vi "Navigation_Main_r0.vi"() -> ()   [LabVIEW 2015]
uses:
  <vilib>/myRIO/Instrument Drivers/Onboard IO/PWM/typedefs/PWM Reference.ctl
  <vilib>/myRIO/Common/Instrument Driver Framework/Utilities/typedefs/myRIO Generic Hardware Reference.ctl
  <vilib>/myRIO/Common/Instrument Driver Framework/Utilities/typedefs/Hardware Version Enum.ctl
  <vilib>/myRIO/Common/Instrument Driver Framework/Utilities/typedefs/myRIO v1.0 Reference.ctl
  <vilib>/myRIO/Common/Instrument Driver Framework/Utilities/typedefs/Generic FPGA Reference.ctl
  <vilib>/myRIO/Common/Instrument Driver Framework/myRIO v1.0/PWM/typedefs/PWM Channels Enum.ctl
  <vilib>/myRIO/Instrument Drivers/Onboard IO/PWM/typedefs/PWM Configuration.ctl
  <vilib>/userdefined/High Color/nirio_resource_hc.ctl
  <vilib>/myRIO/Common/Instrument Driver Framework/myRIO v1.0/PWM/vis/myRIO v1.1 Open PWM.vi
  <vilib>/myRIO/Common/Instrument Driver Framework/Utilities/vis/Validate Channels.vi
  <vilib>/myRIO/Common/Instrument Driver Framework/myRIO v1.0/PWM/vis/myRIO v1.0 Reserve PWM.vi
  <vilib>/myRIO/Instrument Drivers/Onboard IO/PWM/vis/Set Duty Cycle and Frequency.vi
  <vilib>/myRIO/Common/Instrument Driver Framework/myRIO v1.0/PWM/vis/myRIO v1.0 Build MUX Configuration PWM.vi
  <vilib>/myRIO/Common/Instrument Driver Framework/myRIO v1.0/Resource Manager/vis/myRIO v1.0 Reserve Channel List.vi
  <vilib>/myRIO/Common/Instrument Driver Framework/myRIO v1.0/Resource Manager/vis/myRIO v1.0 Create Configuration List.vi
  <vilib>/myRIO/Common/Instrument Driver Framework/myRIO v1.0/Resource Manager/vis/myRIO v1.0 Reserve Channel.vi
  <vilib>/myRIO/Common/Instrument Driver Framework/myRIO v1.0/Resource Manager/vis/myRIO v1.0 Unreserve Channel.vi
  <vilib>/myRIO/Common/Instrument Driver Framework/myRIO v1.0/Resource Manager/vis/myRIO v1.0 Build Mutex Name.vi
  <vilib>/FPGAPlugInAG/myRIO-1900/niLvFpga_Open_myRIO-1900.vi
  <vilib>/rvi/interface/common/dynamic/niFpgaDynamicAddResources.vi
  <vilib>/myRIO/Common/Instrument Driver Framework/Utilities/vis/FPGA Ref Manager.vi
  <vilib>/Utility/error.llb/Error Cluster From Error Code.vi
  <vilib>/myRIO/Common/Instrument Driver Framework/Utilities/vis/Ref Counter.vi
  <vilib>/rvi/errors/niLvFpgaAdjustHostInterfaceError.vi
  <vilib>/Utility/VariantDataType/GetNumericInfo.vi
  <vilib>/myRIO/Common/Instrument Driver Framework/myRIO v1.0/myRIO v1.1 Open.vi
  <vilib>/myRIO/Common/Instrument Driver Framework/Utilities/vis/IO Manager.vi
  <vilib>/myRIO/Common/Instrument Driver Framework/Utilities/vis/Configuration Manager.vi
  <vilib>/myRIO/Common/Instrument Driver Framework/myRIO v1.0/Resource Manager/vis/myRIO v1.0 Configure IO.vi
  <vilib>/myRIO/Common/Instrument Driver Framework/myRIO v1.0/myRIO v1.0 Close.vi
  <vilib>/myRIO/Common/Instrument Driver Framework/myRIO v1.0/PWM/vis/myRIO v1.0 Write PWM.vi
  <vilib>/rvi/interface/nirviOpenFPGA/nirviOpenFPGA.xnode
  Navi/E/FPGA Bitfiles/NavigationProjec_FPGATarget2_FPGAMainNavigati_PWPHW8gwDxI.lvbitx
  <vilib>/rvi/interface/nirviReadWriteControl/nirviReadWriteControl.xnode
  <vilib>/myRIO/Instrument Drivers/Onboard IO/PWM/vis/myRIO PWM Open.xnode
  <vilib>/myRIO/Instrument Drivers/Onboard IO/PWM/PWM.lvlib
  <vilib>/myRIO/Instrument Drivers/Utilities/Utilities.lvlib
  NiFpgaLv.dll
  <vilib>/rvi/interface/Simulation/niFpgaSimulationCallBeginRW.vi
panel:
  out "left rear pwm":dbl
  out "left front pwm":dbl
  out "left mid pwm":dbl
  out "right rear pwm":dbl
  out "right mid pwm":dbl
  out "right front pwm":dbl
  in  "Full Ahead Captain":bool
  out "LF Rot Velocity (rot/s)":dbl
  out "LM Rot Velocity (rot/s)":dbl
  out "LR Rot Velocity (rot/s)":dbl
  in  "All Left Enable":bool
  in  "All Right Enable":bool
  out "RR Rot Velocity (rot/s)":dbl
  out "RM Linear Velocity (rot/s)":dbl
  out "RF Linear Velocity (rot/s)":dbl
  in  "Auto?":bool
  in  "Encoder Reset":bool
  out "L Min Linear Velocity (ft/s) 2":dbl
  out "R Min Linear Velocity (ft/s)  2":dbl
  in  "Goal Y":dbl=3.0 format="%#_13g"
  in  "Goal X":dbl=20.0 format="%#_13g"
  out "x+y":dbl
  in  "Current Y Pos":dbl=5.0 format="%#_13g"
  in  "Current X Pos":dbl=20.0 format="%#_13g"
  out "SYS.SELECTA":u8 format="%08b"
  out "ENC.B_c.CNTR":i32
  out "ENC.B_b.CNTR":i32
  out "ENC.B_a.CNTR":i32
  out "ENC.A_c.CNTR":i32
  out "ENC.A_b.CNTR":i32
  out "ENC.A_a.CNTR":i32
  out "Toggle \nIndicator":bool
  in  "R Desired Input Velocity (ft/s) 2":dbl(knob) scale=-4.0..4.0
  in  "Right Front Enable":bool
  in  "Right Mid Enable":bool
  in  "Right Rear Enable":bool
  in  "Left front enable":bool
  in  "Left mid enable":bool
  in  "Left rear enable":bool
  in  "Sync L -> R":bool
  in  "R Min Linear Velocity (ft/s)":dbl=-2.0 format="%#_13g"
  in  "R Max Linear Velocity (ft/s)":dbl=2.0 format="%#_13g"
  in  "L Min Linear Velocity (ft/s)":dbl=-2.0 format="%#_13g"
  in  "L Max Linear Velocity (ft/s)":dbl=2.0 format="%#_13g"
  out "Current Rot Velocity (rot/s)":T1(graph)
  in  "L Desired Input Velocity (ft/s)":dbl(knob) scale=-4.0..4.0
  # "Motor Control Parameters"
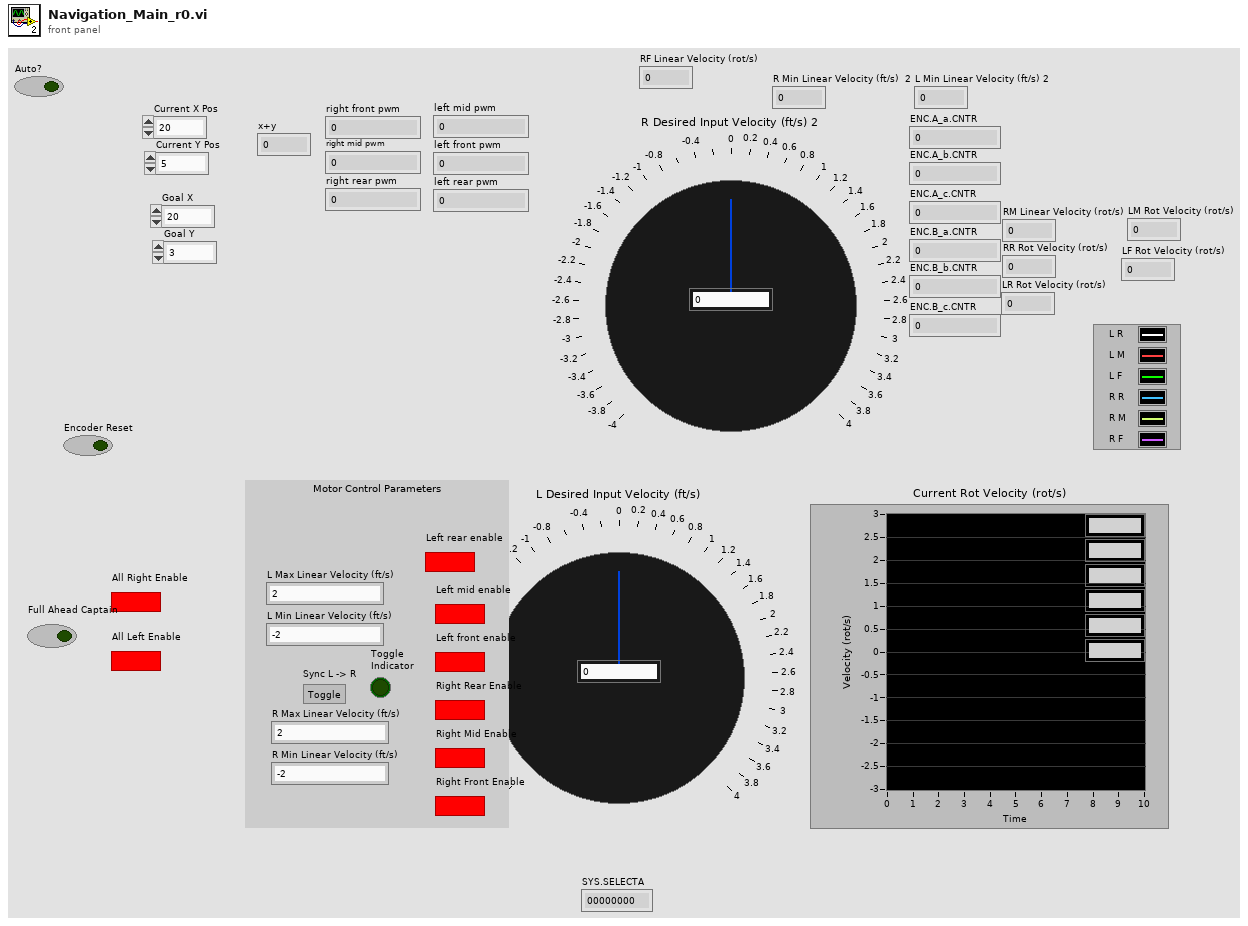
[diagram p1: front panel]
types:
  T1 = cluster{"Rotational Velocity (RPS)":dbl, "Rotational Velocity (RPS)":dbl, "Rotational Velocity (RPS)":dbl, "Rotational Velocity (RPS)":dbl, "Rotational Velocity (RPS)":dbl, "Rotational Velocity (RPS)":dbl}
  T2 = typedef "nirio_resource_hc.ctl" = tag
  T3 = typedef "Hardware Version Enum.ctl" = enum16{"Unknown", "myRIO-1900", "myRIO-1950", "roboRIO"}
  T4 = typedef "PWM.lvlib/PWM Reference.ctl" = cluster{"myRIO Reference":T5, "PWM Channels Enum":T8, "PWM Configuration":T9}
  T5 = typedef "myRIO Generic Hardware Reference.ctl" = cluster{"myRIO Model":T3, "myRIO Hardware Reference":T6}
  T6 = typedef "myRIO v1.0 Reference.ctl" = cluster{"Generic FPGA Reference":T7, "Allow multiple opens":bool}
  T7 = typedef "Generic FPGA Reference.ctl" = refnum<k20>
  T8 = typedef "PWM Channels Enum.ctl" = enum16{"Not Connected", "C/PWM0", "C/PWM1", "A/PWM0", "A/PWM1", "A/PWM2", "B/PWM0", "B/PWM1", "B/PWM2", "PWM/PWM0", "PWM/PWM1", "PWM/PWM2", "PWM/PWM3", "PWM/PWM4", "PWM/PWM5", "PWM/PWM6", "PWM/PWM7", "PWM/PWM8", "PWM/PWM9"}
  T9 = typedef "PWM.lvlib/PWM Configuration.ctl" = cluster{"Frequency":dbl, "Duty Cycle":dbl}
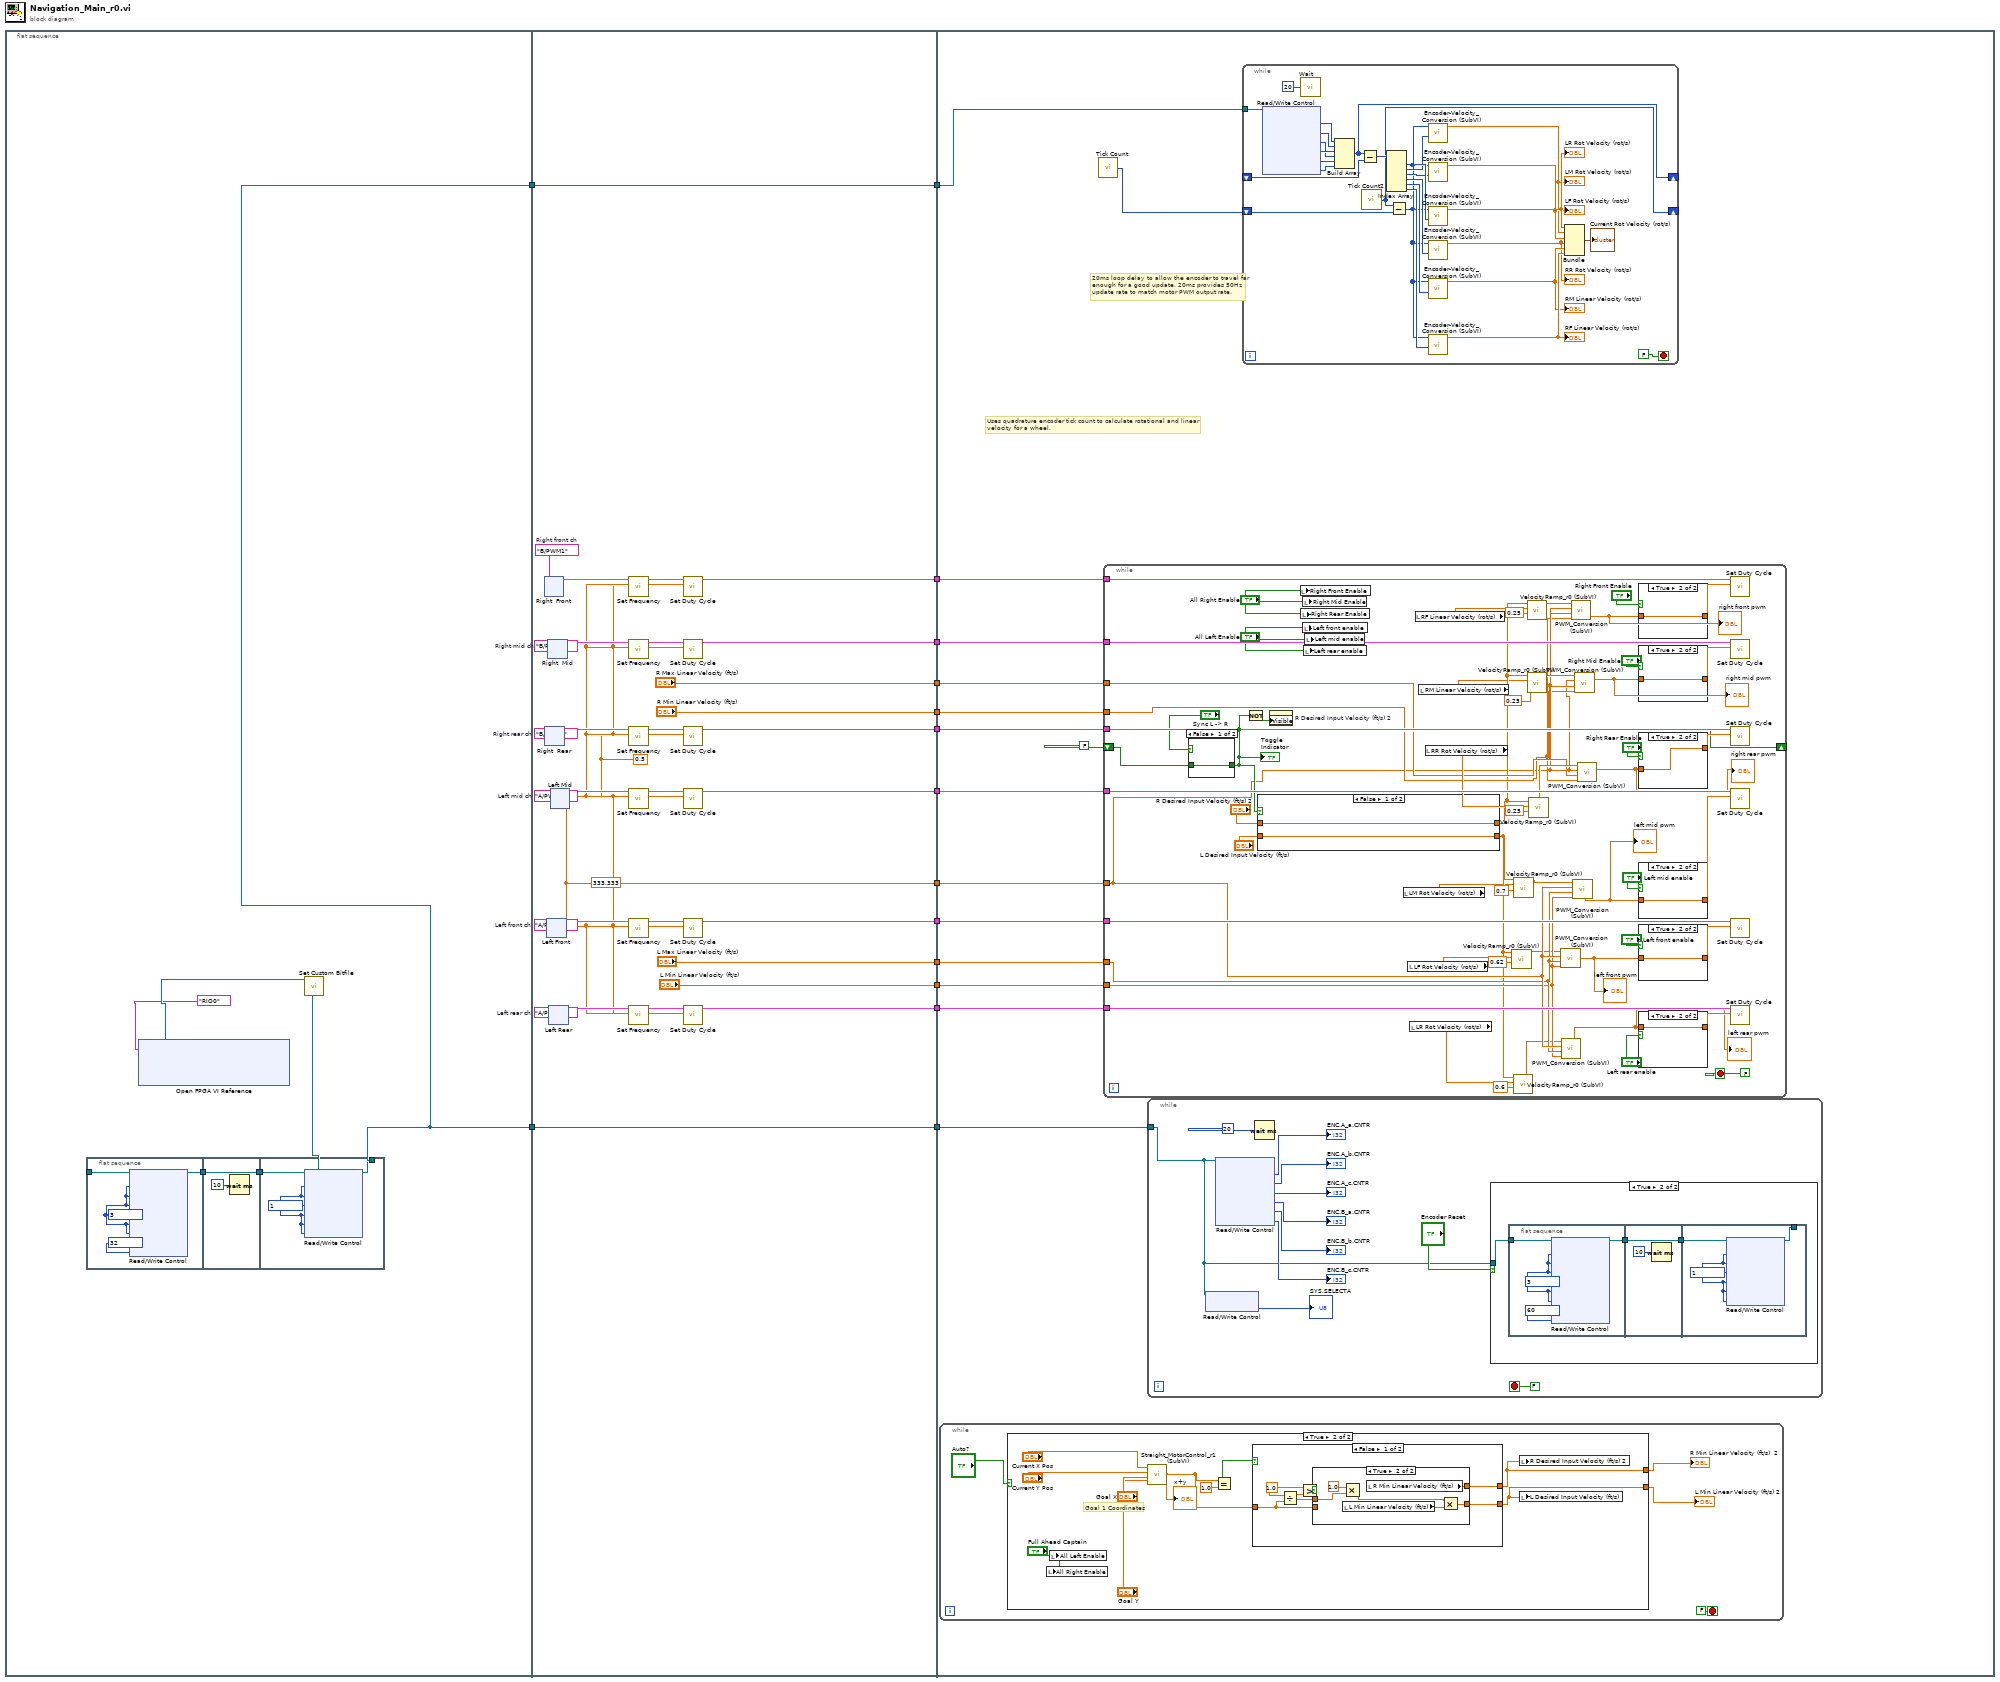
[diagram p0: block diagram]
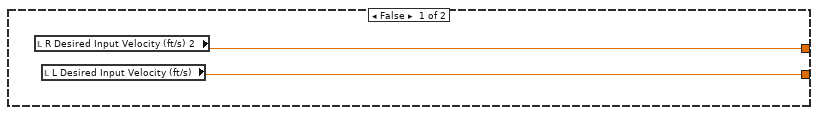
[diagram p2: hidden frame]
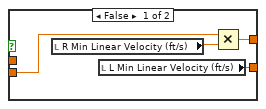
[diagram p3: hidden frame]
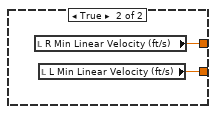
[diagram p4: hidden frame]
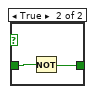
[diagram p6: hidden frame]
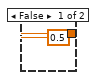
[diagram p7: hidden frame]
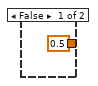
[diagram p8: hidden frame]
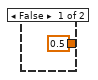
[diagram p9: hidden frame]
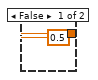
[diagram p10: hidden frame]
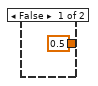
[diagram p11: hidden frame]
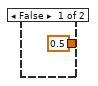
[diagram p12: hidden frame]
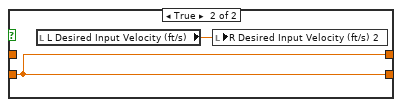
[diagram p13: hidden frame]
diagram:
  n1 = flat-sequence {
    tunnel: [w18] -> w3
    tunnel: [w18] -> w1
    tunnel: [w50] -> w15
    tunnel: [w45] -> w14
    tunnel: [w41] -> w13
    tunnel: [w40] -> w12
    tunnel: [w39] -> w11
    tunnel: [w38] -> w10
    tunnel: [w37] -> w9
    tunnel: ["L Max Linear Velocity (ft/s)"] -> w8
    tunnel: ["L Min Linear Velocity (ft/s)"] -> w7
    tunnel: ["R Max Linear Velocity (ft/s)"] -> w6
    tunnel: ["R Min Linear Velocity (ft/s)"] -> w5
    tunnel: [w32] -> w4
    tunnel: w3 -> [w31]
    tunnel: [w31] -> w2
    tunnel: w1 -> [w32]
    tunnel: w15 -> [w172]
    tunnel: w14 -> [w171]
    tunnel: w13 -> [w170]
    tunnel: w12 -> [w169]
    tunnel: w11 -> [w168]
    tunnel: w10 -> [w167]
    tunnel: w9 -> [w166]
    tunnel: w8 -> [w165]
    tunnel: w7 -> [w164]
    tunnel: w6 -> [w163]
    tunnel: w5 -> [w162]
    tunnel: w4 -> [w160]
    tunnel: w2 -> [w159]
    frame #0 {
      n2 = flat-sequence {
        tunnel: w19 -> [w24]
        tunnel: [w22] -> w21
        tunnel: w21 -> [w26]
        tunnel: [w26] -> w20
        tunnel: w20 -> [w29]
        tunnel: [w28] -> w18
        frame #0 {
          w23 = u8 32 ("SYS.SELECTA")
          w25 = u8 3 ("ENC.B_c.CNFG")
          n3 = xnode "Read/Write Control"("FPGA VI Reference In"=w24, "ENC.A_a.CNFG"=w25, "ENC.A_b.CNFG"=w25, "ENC.A_c.CNFG"=w25, "ENC.B_a.CNFG"=w25, "ENC.B_b.CNFG"=w25, "ENC.B_c.CNFG"=w25, "SYS.SELECTA"=w23, "SYS.SELECTB"=w23) -> ("FPGA VI Reference Out"=w22:refnum<k20>)  [unwired: 1 in, 1 out]
        }
        frame #1 {
          n4 = Wait (ms)(milliseconds to wait=u32 10) -> ()  [unwired: 1 out]
        }
        frame #2 {
          w30 = u8 1 ("ENC.B_c.CNFG")
          n5 = xnode "Read/Write Control"("FPGA VI Reference In"=w29, "ENC.A_a.CNFG"=w30, "ENC.A_b.CNFG"=w30, "ENC.A_c.CNFG"=w30, "ENC.B_a.CNFG"=w30, "ENC.B_b.CNFG"=w30, "ENC.B_c.CNFG"=w30) -> ("FPGA VI Reference Out"=w28:refnum<k20>)  [unwired: 1 in, 1 out]
        }
      }
      n6 = xnode "Open FPGA VI Reference"("resource name"=tag "RIO0") -> ("FPGA VI Reference Out"=w17:refnum<k20>)  [unwired: 1 in, 1 out]
      n7 = call <vilib>:"Set Custom Bitfile.vi"("Custom FPGA Reference In"=w17) -> ("Custom FPGA Reference Out"=w19:refnum<k20>)  [unwired: 9 in, 1 out]
    }
    frame #1 {
      w42 = 0.5 ("Duty Cycle")
      w50 = 333.333 ("Frequency [Hz]")
      w57 = tag "B/PWM2"  # Right rear ch
      w58 = tag "B/PWM0"  # Right mid ch
      w59 = tag "B/PWM1"  # Right front ch
      w60 = tag "A/PWM2"  # Left rear ch
      w61 = tag "A/PWM1"  # Left mid ch
      w62 = tag "A/PWM0"  # Left front ch
      n8 = xnode "Right  Front"("Channel Name"=w59) -> ("PWM Ref Out"=w53:T4)  [unwired: 2 in, 1 out]
      n9 = xnode "Right  Rear"("Channel Name"=w57) -> ("PWM Ref Out"=w51:T4)  [unwired: 2 in, 1 out]
      n10 = xnode "Left Front"("Channel Name"=w62) -> ("PWM Ref Out"=w56:T4)  [unwired: 2 in, 1 out]
      n11 = xnode "Right  Mid"("Channel Name"=w58) -> ("PWM Ref Out"=w52:T4)  [unwired: 2 in, 1 out]
      n12 = xnode "Left Rear"("Channel Name"=w60) -> ("PWM Ref Out"=w54:T4)  [unwired: 2 in, 1 out]
      n13 = xnode "Left Mid"("Channel Name"=w61) -> ("PWM Ref Out"=w55:T4)  [unwired: 2 in, 1 out]
      n14 = call <vilib>:"Set Frequency.vi"("Frequency [Hz]"=w50, "PWM Ref In"=w53) -> ("PWM Ref Out"=w46:T4)  [unwired: 7 in, 1 out]
      n15 = call <vilib>:"Set Frequency.vi"("Frequency [Hz]"=w50, "PWM Ref In"=w52) -> ("PWM Ref Out"=w47:T4)  [unwired: 7 in, 1 out]
      n16 = call <vilib>:"Set Frequency.vi"("Frequency [Hz]"=w50, "PWM Ref In"=w51) -> ("PWM Ref Out"=w48:T4)  [unwired: 7 in, 1 out]
      n17 = call <vilib>:"Set Frequency.vi"("Frequency [Hz]"=w50, "PWM Ref In"=w55) -> ("PWM Ref Out"=w43:T4)  [unwired: 7 in, 1 out]
      n18 = call <vilib>:"Set Frequency.vi"("Frequency [Hz]"=w50, "PWM Ref In"=w56) -> ("PWM Ref Out"=w49:T4)  [unwired: 7 in, 1 out]
      n19 = call <vilib>:"Set Frequency.vi"("Frequency [Hz]"=w50, "PWM Ref In"=w54) -> ("PWM Ref Out"=w44:T4)  [unwired: 7 in, 1 out]
      n20 = call <vilib>:"Set Duty Cycle.vi"("Duty Cycle"=w42, "PWM Ref In"=w46) -> ("PWM Ref Out"=w41:T4)  [unwired: 7 in, 1 out]
      n21 = call <vilib>:"Set Duty Cycle.vi"("Duty Cycle"=w42, "PWM Ref In"=w47) -> ("PWM Ref Out"=w40:T4)  [unwired: 7 in, 1 out]
      n22 = call <vilib>:"Set Duty Cycle.vi"("Duty Cycle"=w42, "PWM Ref In"=w48) -> ("PWM Ref Out"=w39:T4)  [unwired: 7 in, 1 out]
      n23 = call <vilib>:"Set Duty Cycle.vi"("Duty Cycle"=w42, "PWM Ref In"=w43) -> ("PWM Ref Out"=w38:T4)  [unwired: 7 in, 1 out]
      n24 = call <vilib>:"Set Duty Cycle.vi"("Duty Cycle"=w42, "PWM Ref In"=w49) -> ("PWM Ref Out"=w37:T4)  [unwired: 7 in, 1 out]
      n25 = call <vilib>:"Set Duty Cycle.vi"("Duty Cycle"=w42, "PWM Ref In"=w44) -> ("PWM Ref Out"=w45:T4)  [unwired: 7 in, 1 out]
    }
    frame #2 {
      # "Uses quadrature encoder tick count to calculate rotational and linear velocity for a wheel."
      # "20ms loop delay to allow the encoder to travel far enough for a good update. 20ms provides 50Hz update rate to match motor PWM output rate."
      n26 = while {
        stop <- FALSE stop-if-true
        n27 = case shown="True" "Auto?" {
          tunnel: [w178 w181] -> w176
          tunnel: [w179 w182] -> w175
          frame False {
            n28 = local read "R Desired Input Velocity (ft/s) 2"() -> (w178:dbl)
            n29 = local read "L Desired Input Velocity (ft/s)"() -> (w179:dbl)
          }
          frame True {
            # "Goal 1 Coordinates"
            n30 = local write "All Right Enable"("Full Ahead Captain") -> ()
            n31 = local write "All Left Enable"("Full Ahead Captain") -> ()
            n32 = call "Straight_MotorControl_r1 (SubVI).vi"("Goal Y Coord"="Goal Y", "Goal X Coord"="Goal X", "Current Y Pos"="Current Y Pos", "Current X Pos"="Current X Pos") -> ("Numeric Out Y"=w187:dbl)  [unwired: 6 in, 1 out]
            "x+y" <- w187
            n33 = Equal?(x=w187, y=1.0) -> (x = y?=w185:bool)
            n34 = case shown="False" w185 {
              tunnel: [w192 w206] -> w182
              tunnel: [w191 w207] -> w181
              tunnel: w187 -> [w190 _]
              frame False {
                w195 = 1.0 ("x")
                n35 = Divide(x=w195, y=w190) -> (x/y=w194:dbl)
                n36 = Greater?(x=w195, y=w194) -> (0:w193:bool)
                n37 = case shown="True" w193 {
                  tunnel: w194 -> [_ w202]
                  tunnel: [w196 w203] -> w192
                  tunnel: [w197 w204] -> w191
                  tunnel: w190 -> [w199 _]
                  frame False {
                    n38 = local read "R Min Linear Velocity (ft/s)"() -> (w198:dbl)
                    n39 = local read "L Min Linear Velocity (ft/s)"() -> (w196:dbl)
                    n40 = Multiply(x=w199, y=w198) -> (x*y=w197:dbl)
                  }
                  frame True {
                    n41 = local read "L Min Linear Velocity (ft/s)"() -> (w205:dbl)
                    n42 = Multiply(x=1.0, y=w202) -> (x*y=w201:dbl)
                    n43 = local read "R Min Linear Velocity (ft/s)"() -> (w204:dbl)
                    n44 = Multiply(x=w201, y=w205) -> (x*y=w203:dbl)
                  }
                }
              }
              frame True {
                n45 = local read "R Min Linear Velocity (ft/s)"() -> (w207:dbl)
                n46 = local read "L Min Linear Velocity (ft/s)"() -> (w206:dbl)
              }
            }
            n47 = local write "R Desired Input Velocity (ft/s) 2"(w181) -> ()
            n48 = local write "L Desired Input Velocity (ft/s)"(w182) -> ()
          }
        }
        "R Min Linear Velocity (ft/s)  2" <- w176
        "L Min Linear Velocity (ft/s) 2" <- w175
      }
      n49 = call "Tick Count"() -> ("Tick Count(uSec)"=w173:u32)
      n50 = while {
        tunnel: w172 -> [w250]
        tunnel: w171 -> [w277]
        tunnel: w170 -> [w282]
        tunnel: w169 -> [w281]
        tunnel: w168 -> [w280]
        tunnel: w167 -> [w279]
        tunnel: w166 -> [w278]
        tunnel: w165 -> [w249]
        tunnel: w164 -> [w248]
        tunnel: w163 -> [w260]
        tunnel: w162 -> [w259]
        shift-right: [w266] -> _
        shift-left: FALSE -> [w267]
        stop <- FALSE stop-if-true
        n51 = case shown="False" "Sync L -> R" {
          tunnel: w267 -> [w289 w291]
          tunnel: [w289 w290] -> w266
          frame False {
          }
          frame True {
            n52 = Not(x=w291) -> (.not. x?=w290:bool)
          }
        }
        "Toggle \nIndicator" <- w266
        n53 = Not(x=w266) -> (.not. x?=w269:bool)
        n54 = case shown="False" w266 {
          tunnel: "L Desired Input Velocity (ft/s)" -> [w305 w306]
          tunnel: [w305 w306] -> w245
          tunnel: "R Desired Input Velocity (ft/s) 2" -> [w304 _]
          tunnel: [w304 w306] -> w258
          frame False {
          }
          frame True {
            n55 = local read "L Desired Input Velocity (ft/s)"() -> (w307:dbl)
            n56 = local write "R Desired Input Velocity (ft/s) 2"(w307) -> ()
          }
        }
        n57 = property on="R Desired Input Velocity (ft/s) 2" class="Knob (strict)"("Visible"=w269) -> ()  [unwired: 2 in, 2 out]
        n58 = local write "Right Front Enable"("All Right Enable") -> ()
        n59 = local write "Right Rear Enable"("All Right Enable") -> ()
        n60 = local write "Right Mid Enable"("All Right Enable") -> ()
        n61 = local write "Left front enable"("All Left Enable") -> ()
        n62 = local write "Left rear enable"("All Left Enable") -> ()
        n63 = local write "Left mid enable"("All Left Enable") -> ()
        n64 = local read "LM Rot Velocity (rot/s)"() -> (w244:dbl)
        n65 = local read "LF Rot Velocity (rot/s)"() -> (w252:dbl)
        n66 = local read "LR Rot Velocity (rot/s)"() -> (w251:dbl)
        n67 = local read "RF Linear Velocity (rot/s)"() -> (w256:dbl)
        n68 = local read "RM Linear Velocity (rot/s)"() -> (w257:dbl)
        n69 = local read "RR Rot Velocity (rot/s)"() -> (w263:dbl)
        n70 = call "VelocityRamp_r0 (SubVI).vi"("Step Size"=0.62, "Current Velocity (RPS)"=w252, "Input Velocity (RPS)"=w245) -> ("Output Velocity (RPS)"=w246:dbl)  [unwired: 8 in]
        n71 = call "VelocityRamp_r0 (SubVI).vi"("Step Size"=0.6, "Current Velocity (RPS)"=w251, "Input Velocity (RPS)"=w245) -> ("Output Velocity (RPS)"=w247:dbl)  [unwired: 8 in]
        n72 = call "VelocityRamp_r0 (SubVI).vi"("Step Size"=0.7, "Current Velocity (RPS)"=w244, "Input Velocity (RPS)"=w245) -> ("Output Velocity (RPS)"=w243:dbl)  [unwired: 8 in]
        n73 = call "VelocityRamp_r0 (SubVI).vi"("Step Size"=0.25, "Current Velocity (RPS)"=w256, "Input Velocity (RPS)"=w258) -> ("Output Velocity (RPS)"=w261:dbl)  [unwired: 8 in]
        n74 = call "VelocityRamp_r0 (SubVI).vi"("Step Size"=0.25, "Current Velocity (RPS)"=w257, "Input Velocity (RPS)"=w258) -> ("Output Velocity (RPS)"=w262:dbl)  [unwired: 8 in]
        n75 = call "VelocityRamp_r0 (SubVI).vi"("Step Size"=0.25, "Current Velocity (RPS)"=w263, "Input Velocity (RPS)"=w258) -> ("Output Velocity (RPS)"=w264:dbl)  [unwired: 8 in]
        n76 = call "PWM_Conversion (SubVI).vi"("Min Linear Velocity (ft/s)"=w248, "Max Linear Velocity (ft/s)"=w249, "PWM Frequency"=w250, "Linear Velocity Input (ft/s)"=w246) -> ("PWM Signal Output"=w232:dbl)  [unwired: 7 in]
        "left front pwm" <- w232
        n77 = call "PWM_Conversion (SubVI).vi"("Min Linear Velocity (ft/s)"=w248, "Max Linear Velocity (ft/s)"=w249, "PWM Frequency"=w250, "Linear Velocity Input (ft/s)"=w247) -> ("PWM Signal Output"=w233:dbl)  [unwired: 7 in]
        "left rear pwm" <- w233
        n78 = call "PWM_Conversion (SubVI).vi"("Min Linear Velocity (ft/s)"=w259, "Max Linear Velocity (ft/s)"=w260, "PWM Frequency"=w250, "Linear Velocity Input (ft/s)"=w261) -> ("PWM Signal Output"=w234:dbl)  [unwired: 7 in]
        "right front pwm" <- w234
        n79 = call "PWM_Conversion (SubVI).vi"("Min Linear Velocity (ft/s)"=w248, "Max Linear Velocity (ft/s)"=w249, "PWM Frequency"=w250, "Linear Velocity Input (ft/s)"=w243) -> ("PWM Signal Output"=w231:dbl)  [unwired: 7 in]
        "left mid pwm" <- w231
        n80 = call "PWM_Conversion (SubVI).vi"("Min Linear Velocity (ft/s)"=w259, "Max Linear Velocity (ft/s)"=w260, "PWM Frequency"=w250, "Linear Velocity Input (ft/s)"=w262) -> ("PWM Signal Output"=w235:dbl)  [unwired: 7 in]
        "right mid pwm" <- w235
        n81 = call "PWM_Conversion (SubVI).vi"("Min Linear Velocity (ft/s)"=w259, "Max Linear Velocity (ft/s)"=w260, "PWM Frequency"=w250, "Linear Velocity Input (ft/s)"=w264) -> ("PWM Signal Output"=w236:dbl)  [unwired: 7 in]
        "right rear pwm" <- w236
        n82 = case shown="True" "Right Front Enable" {
          tunnel: [0.5 w303] -> w271
          tunnel: w234 -> [_ w303]
          frame False {
          }
          frame True {
          }
        }
        n83 = case shown="True" "Right Mid Enable" {
          tunnel: [0.5 w301] -> w272
          tunnel: w235 -> [_ w301]
          frame False {
          }
          frame True {
          }
        }
        n84 = case shown="True" "Right Rear Enable" {
          tunnel: [0.5 w299] -> w273
          tunnel: w236 -> [_ w299]
          frame False {
          }
          frame True {
          }
        }
        n85 = case shown="True" "Left mid enable" {
          tunnel: [0.5 w297] -> w274
          tunnel: w231 -> [_ w297]
          frame False {
          }
          frame True {
          }
        }
        n86 = case shown="True" "Left front enable" {
          tunnel: [0.5 w295] -> w275
          tunnel: w232 -> [_ w295]
          frame False {
          }
          frame True {
          }
        }
        n87 = case shown="True" "Left rear enable" {
          tunnel: [0.5 w293] -> w276
          tunnel: w233 -> [_ w293]
          frame False {
          }
          frame True {
          }
        }
        n88 = call <vilib>:"Set Duty Cycle.vi"("Duty Cycle"=w271, "PWM Ref In"=w282) -> ()  [unwired: 7 in, 2 out]
        n89 = call <vilib>:"Set Duty Cycle.vi"("Duty Cycle"=w272, "PWM Ref In"=w281) -> ()  [unwired: 7 in, 2 out]
        n90 = call <vilib>:"Set Duty Cycle.vi"("Duty Cycle"=w273, "PWM Ref In"=w280) -> ()  [unwired: 7 in, 2 out]
        n91 = call <vilib>:"Set Duty Cycle.vi"("Duty Cycle"=w274, "PWM Ref In"=w279) -> ()  [unwired: 7 in, 2 out]
        n92 = call <vilib>:"Set Duty Cycle.vi"("Duty Cycle"=w275, "PWM Ref In"=w278) -> ()  [unwired: 7 in, 2 out]
        n93 = call <vilib>:"Set Duty Cycle.vi"("Duty Cycle"=w276, "PWM Ref In"=w277) -> ()  [unwired: 7 in, 2 out]
      }
      n94 = while {
        tunnel: w160 -> [w208]
        stop <- FALSE stop-if-true
        n95 = xnode "Read/Write Control"("FPGA VI Reference In"=w208) -> ("SYS.SELECTA"=→"SYS.SELECTA":u8)  [unwired: 1 in, 2 out]
        n96 = xnode "Read/Write Control"("FPGA VI Reference In"=w208) -> ("ENC.A_a.CNTR"=→"ENC.A_a.CNTR":u32, "ENC.A_b.CNTR"=→"ENC.A_b.CNTR":u32, "ENC.A_c.CNTR"=→"ENC.A_c.CNTR":u32, "ENC.B_a.CNTR"=→"ENC.B_a.CNTR":u32, "ENC.B_b.CNTR"=→"ENC.B_b.CNTR":u32, "ENC.B_c.CNTR"=→"ENC.B_c.CNTR":u32)  [unwired: 1 in, 2 out]
        n97 = Wait (ms)(milliseconds to wait=u32 20) -> ()  [unwired: 1 out]
        n98 = case shown="True" "Encoder Reset" {
          tunnel: w208 -> [_ w219]
          frame False {
          }
          frame True {
            n99 = flat-sequence {
              tunnel: w219 -> [w224]
              tunnel: [w222] -> w221
              tunnel: w221 -> [w226]
              tunnel: [w226] -> w220
              tunnel: w220 -> [w229]
              tunnel: [w228] -> _
              frame #0 {
                w223 = u8 60 ("SYS.SELECTA")
                w225 = u8 3 ("ENC.B_c.CNFG")
                n100 = xnode "Read/Write Control"("FPGA VI Reference In"=w224, "ENC.A_a.CNFG"=w225, "ENC.A_b.CNFG"=w225, "ENC.A_c.CNFG"=w225, "ENC.B_a.CNFG"=w225, "ENC.B_b.CNFG"=w225, "ENC.B_c.CNFG"=w225, "SYS.SELECTA"=w223, "SYS.SELECTB"=w223) -> ("FPGA VI Reference Out"=w222:refnum<k20>)  [unwired: 1 in, 1 out]
              }
              frame #1 {
                n101 = Wait (ms)(milliseconds to wait=u32 10) -> ()  [unwired: 1 out]
              }
              frame #2 {
                w230 = u8 1 ("ENC.B_c.CNFG")
                n102 = xnode "Read/Write Control"("FPGA VI Reference In"=w229, "ENC.A_a.CNFG"=w230, "ENC.A_b.CNFG"=w230, "ENC.A_c.CNFG"=w230, "ENC.B_a.CNFG"=w230, "ENC.B_b.CNFG"=w230, "ENC.B_c.CNFG"=w230) -> ("FPGA VI Reference Out"=w228:refnum<k20>)  [unwired: 1 in, 1 out]
              }
            }
          }
        }
      }
      n103 = while {
        shift-right: [w326] -> _
        shift-left: _ -> [w325]
        shift-right: [w323] -> _
        shift-left: w173 -> [w322]
        tunnel: w159 -> [w333]
        stop <- FALSE stop-if-true
        n104 = xnode "Read/Write Control"("FPGA VI Reference In"=w333) -> ("ENC.A_a.CNTR"=w332:u32, "ENC.A_b.CNTR"=w331:u32, "ENC.A_c.CNTR"=w330:u32, "ENC.B_a.CNTR"=w329:u32, "ENC.B_b.CNTR"=w328:u32, "ENC.B_c.CNTR"=w327:u32)  [unwired: 1 in, 2 out]
        n105 = call "Wait"("Count(mSec)"=u32 20) -> ()  [unwired: 1 out]
        n106 = Build Array(w332, w331, w330, w329, w328, w327) -> (w326:u32[])
        n107 = Subtract(x=w326, y=w325) -> (x-y=w324:u32[])
        n108 = call "Tick Count2"() -> ("Tick Count(uSec)"=w323:u32)
        n109 = Index Array(array=w324) -> (element #1=w321:u32, element #2=w320:u32, element #3=w319:u32, element #4=w318:u32, element #5=w317:u32, element #6=w316:u32)  [unwired: 6 in]
        n110 = Subtract(x=w323, y=w322) -> (x-y=w315:u32)
        n111 = call "Encoder-Velocity_Conversion (SubVI).vi"("delta  Encoder Count"=w320, "dt (uSec)"=w315) -> ("Rotational Velocity (RPS)"=w310:dbl)  [unwired: 7 in, 2 out]
        "LM Rot Velocity (rot/s)" <- w310
        n112 = call "Encoder-Velocity_Conversion (SubVI).vi"("delta  Encoder Count"=w319, "dt (uSec)"=w315) -> ("Rotational Velocity (RPS)"=w309:dbl)  [unwired: 7 in, 2 out]
        "LF Rot Velocity (rot/s)" <- w309
        n113 = call "Encoder-Velocity_Conversion (SubVI).vi"("delta  Encoder Count"=w321, "dt (uSec)"=w315) -> ("Rotational Velocity (RPS)"=w311:dbl)  [unwired: 7 in, 2 out]
        "LR Rot Velocity (rot/s)" <- w311
        n114 = call "Encoder-Velocity_Conversion (SubVI).vi"("delta  Encoder Count"=w318, "dt (uSec)"=w315) -> ("Rotational Velocity (RPS)"=w308:dbl)  [unwired: 7 in, 2 out]
        "RR Rot Velocity (rot/s)" <- w308
        n115 = call "Encoder-Velocity_Conversion (SubVI).vi"("delta  Encoder Count"=w317, "dt (uSec)"=w315) -> ("Rotational Velocity (RPS)"=w312:dbl)  [unwired: 7 in, 2 out]
        "RM Linear Velocity (rot/s)" <- w312
        n116 = call "Encoder-Velocity_Conversion (SubVI).vi"("delta  Encoder Count"=w316, "dt (uSec)"=w315) -> ("Rotational Velocity (RPS)"=w313:dbl)  [unwired: 7 in, 2 out]
        "RF Linear Velocity (rot/s)" <- w313
        n117 = Bundle("Rotational Velocity (RPS)"=w311, "Rotational Velocity (RPS)"=w310, "Rotational Velocity (RPS)"=w309, "Rotational Velocity (RPS)"=w308, "Rotational Velocity (RPS)"=w312, "Rotational Velocity (RPS)"=w313) -> (→"Current Rot Velocity (rot/s)":T1)  [unwired: 1 in]
      }
    }
  }
